vi "SysDef.Property.Remove.vi"(8 "error in (no error)":errorcluster, 10 "Property Name":string, 11 "nodeID":u64) -> (0 "error out":errorcluster, 1 "Removed":bool, 3 "nodeID out":u64)   [LabVIEW 2015, in "System Definition Utilities.lvlib"]
uses:
  System Definition Utilities.lvlib
  NationalInstruments.VeriStand.SystemDefinitionAPI
  <vilib>/NI Veristand/Custom Device API/Custom Device API.lvlib
  NationalInstruments.VeriStand.SystemStorage
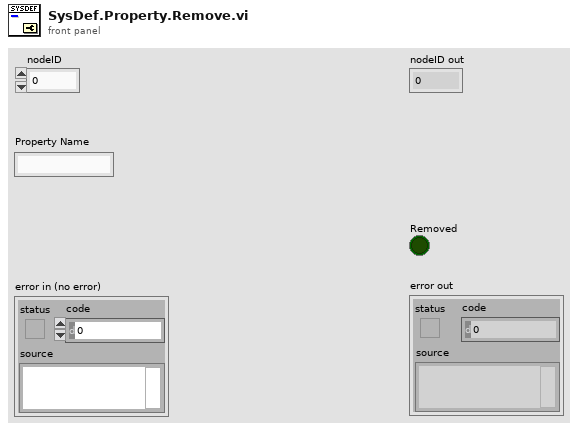
[diagram p1: front panel]
types:
  T1 = typedef "Custom Device API.lvlib/Custom Device Item Ref.ctl" = u64
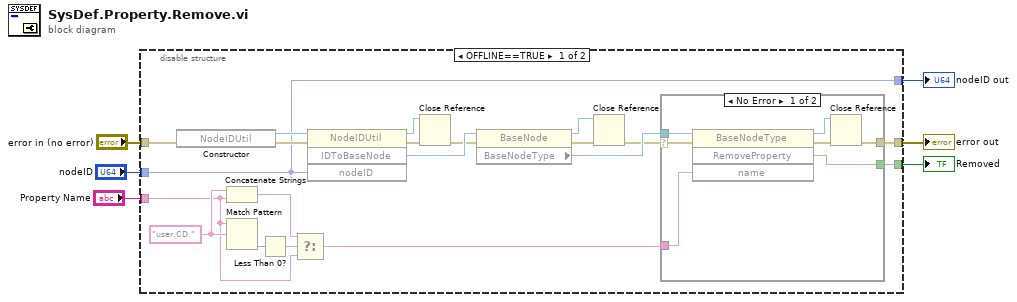
[diagram p0: block diagram]
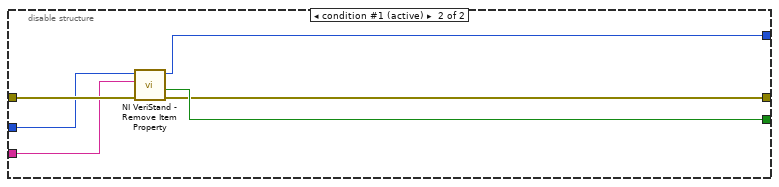
[diagram p3: hidden frame]
diagram:
  n1 = disable-structure shown="OFFLINE==TRUE" {
    disable-tunnel: "Property Name" -> [w8 w38]
    disable-tunnel: [w26 w36] -> w5
    disable-tunnel: [w25 w37] -> w4
    disable-tunnel: "error in (no error)" -> [w22 w40]
    disable-tunnel: "nodeID" -> [w13 w39]
    disable-tunnel: [w13 w35] -> w1
    frame condition #0 {
      w9 = "user.CD." ("regular expression")
      n2 = constructor class="NodeIDUtil"(error in=w22) -> (reference out=w24:refnum<k24>, error out=w23:errorcluster)  [unwired: 2 in, 1 out]
      n3 = Concatenate Strings(w9, w8) -> (w10:string)
      n4 = Match Pattern(string=w8, regular expression=w9) -> (offset past match=w12:i32)  [unwired: 1 in, 3 out]
      n5 = Less Than 0?(x=w12) -> (x < 0?=w11:bool)
      n6 = Select(t=w10, s=w11, f=w8) -> (s? t:f=w7:string)
      n7 = invoke class="NodeIDUtil" method="IDToBaseNode"(reference=w24, error in=w23, "nodeID"=w13) -> (reference out=w16:refnum<k24>, error out=w15:errorcluster, "IDToBaseNode"=w21:refnum<k24>)  [unwired: 1 in, 1 out]
      n8 = Close Reference(reference=w16, error in (no error)=w15) -> (error out=w14:errorcluster)
      n9 = property class="BaseNode"(reference=w21, error in=w14) -> (reference out=w19:refnum<k24>, error out=w18:errorcluster, "BaseNodeType"=w20:refnum<k24>)
      n10 = Close Reference(reference=w19, error in (no error)=w18) -> (error out=w17:errorcluster)
      n11 = case shown="No Error" w17 {
        selector: w17 -> [w32 w34]
        tunnel: w20 -> [w33 _]
        tunnel: w7 -> [w29 _]
        tunnel: [w28 w34] -> w26
        tunnel: [w27 _] -> w25
        frame No Error {
          n12 = invoke class="BaseNodeType" method="RemoveProperty"(reference=w33, error in=w32, "name"=w29) -> (reference out=w30:refnum<k24>, error out=w31:errorcluster, "RemoveProperty"=w27:bool)  [unwired: 1 in, 1 out]
          n13 = Close Reference(reference=w30, error in (no error)=w31) -> (error out=w28:errorcluster)
        }
        frame Error {
        }
      }
    }
    frame condition #1 (active) {
      n14 = call <vilib>:"NI VeriStand - Remove Item Property.vi"("error in (no error)"=w40, "Property Name"=w38, "Item Ref in"=w39) -> ("error out"=w36:errorcluster, "Removed"=w37:bool, "Item Ref out"=w35:T1)  [unwired: 6 in]
    }
  }
  "nodeID out" <- w1
  "error out" <- w5
  "Removed" <- w4
